vi "Hang.vi"(10 "Driver Hang":bool) -> (2 "Hang Voltage":dbl)   [LabVIEW 2016]
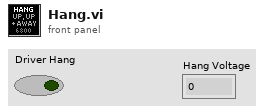
[diagram p1: front panel]
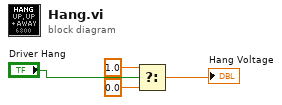
[diagram p0: block diagram]
diagram:
  n1 = Select(t=1.0, s="Driver Hang", f=0.0) -> (s? t:f=→"Hang Voltage":dbl)
